vi "1B calc wind acceleration.vi"(8 "Sail Position":dbl, 9 "time elapsed since last iteration":dbl, 10 "Apparent Wind Speed in":T2, 11 "Absolute Wind\nDirection":T1) -> (3 "Wind dV":T2)   [LabVIEW 2011]
doc: "Calculates velocity from the wind. Uses the apparent wind direction and sail angle to determine the fraction of the wind speed we can go at, using several equations that roughly model boat speed, and then multiplies the wind speed by that fraction.\nTODO: currently only does acceleration in the forward direction. should be upgraded to have a side force as well, which can be balanced by a hydrodynamic side force."
uses:
  2-Think/2 Typedefs/apparent wind speed.ctl
  2-Think/2 Typedefs/apparent wind direction.ctl
  2-Think/2 Typedefs/heading.ctl
  2-Think/2 Globals/2 TuningConstants.vi
  2-Think/2 Globals/2 Global.vi
panel:
  out "In Irons?":bool
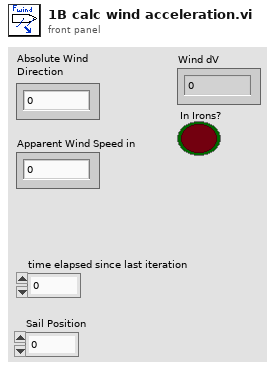
[diagram p1: front panel]
types:
  T1 = typedef "apparent wind direction.ctl" = dbl
  T2 = typedef "apparent wind speed.ctl" = dbl
  T3 = typedef "heading.ctl" = dbl
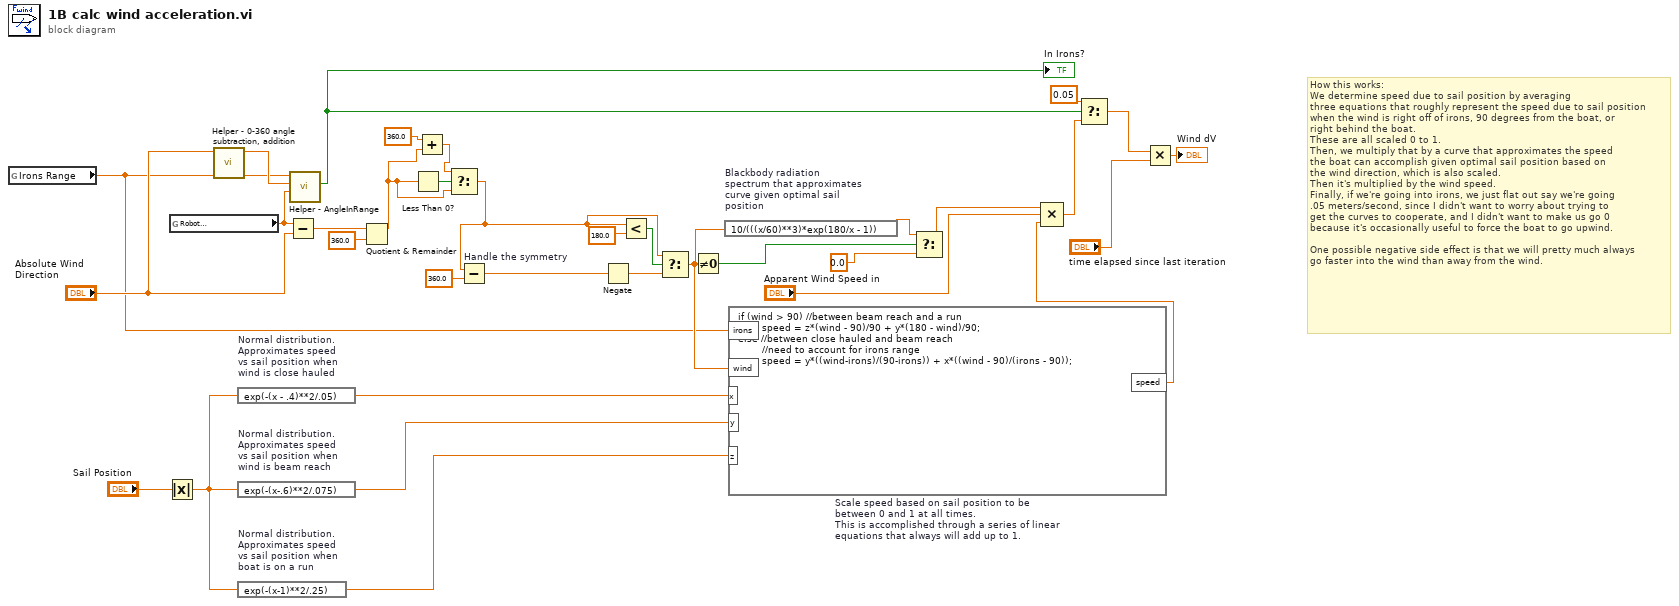
[diagram p0: block diagram]
diagram:
  # "How this works:\nWe determine speed due to sail position by averaging\nthree equations that roughly represent the speed due to sail position\nwhen the wind is right off of irons, 90 degrees from the boat, or\nright behind the boat.\nThese are all scaled 0 to 1.\nThen, we multiply that by a curve that approximates the speed\nthe boat can accomplish given optimal sail position based on\nthe wind direction, which is also scaled.\nThen it's multiplied by the wind speed.\nFinally, if we're going into irons, we just flat out say we're going\n.05 meters/second, since I didn't want to worry about trying to\nget the curves to cooperate, and I didn't want to make us go 0\nbecause it's occasionally useful to force the boat to go upwind.\n\nOne possible negative side effect is that we will pretty much always\ngo faster into the wind than away from the wind."
  n1 = global read "2 TuningConstants.vi" "Irons Range"() -> (w5:dbl)
  n2 = Absolute Value(x="Sail Position") -> (abs(x)=w1:dbl)
  n3 = global read "2 Global.vi" "Robot\nHeading"() -> (w15:T3)
  n4 = call "Helper - 0-360 angle subtraction, addition.vi"("y"=w5, "x"="Absolute Wind\nDirection") -> ("x + y"=w3:dbl, "x - y"=w4:T1)  [unwired: 8 in]
  n5 = expression code="exp(-(x - .4)**2/.05)" "Normal distribution.\nApproximates speed \nvs sail position when\nwind is close hauled"(w1) -> (w24:dbl)
  n6 = expression code="exp(-(x-.6)**2/.075)" "Normal distribution.\nApproximates speed\nvs sail position when\nwind is beam reach"(w1) -> (w23:dbl)
  n7 = expression code="exp(-(x-1)**2/.25)" "Normal distribution.\nApproximates speed\nvs sail position when\nboat is on a run"(w1) -> (w22:dbl)
  n8 = Subtract(x=w15, y="Absolute Wind\nDirection") -> (x-y=w12:T3)
  n9 = call "Helper - AngleInRange.vi"("Angle to check"=w15, "Angle 2"=w4, "Angle 1"=w3) -> ("In range?"=w14:bool)  [unwired: 8 in]
  "In Irons?" <- w14
  n10 = Quotient & Remainder(x=w12, y=T3 360.0) -> (x-y*floor(x/y)=w7:T3)  [unwired: 1 out]
  n11 = Less Than 0?(x=w7) -> (x < 0?=w10:bool)
  n12 = Add(x=T3 360.0, y=w7) -> (x+y=w8:T3)
  n13 = Select(t=w8, s=w10, f=w7) -> (s? t:f=w9:T3)
  n14 = Subtract "Handle the symmetry"(x=w9, y=T1 360.0) -> (x-y=w25:T3)
  n15 = Negate(x=w25) -> (-x=w26:T3)
  n16 = Less?(x=w9, y=T1 180.0) -> (x < y?=w28:bool)
  n17 = Select(t=w9, s=w28, f=w26) -> (s? t:f=w17:T3)
  n18 = Not Equal To 0?(x=w17) -> (x != 0?=w16:bool)
  n19 = expression code="10/(((x/60)**3)*exp(180/x - 1))" "Blackbody radiation\nspectrum that approximates\ncurve given optimal sail\nposition"(w17) -> (w20:T3)
  n20 = formula code="if (wind > 90) //between beam reach and a run\n        speed = z*(wind - 90)/90 + y*(180 - wind)/90;\nelse //between close hauled and beam reach\n        //need to account for irons range\n        speed = y*((wind-irons)/(90-irons)) + x*((wind - 90)/(irons - 90));" "Scale speed based on sail position to be between 0 and 1 at all times.\nThis is accomplished through a series of linear equations that always will add up to 1."("x"=w24, "y"=w23, "z"=w22, "wind"=w17, "irons"=w5) -> ("speed"=w21:dbl)
  n21 = Select(t=w20, s=w16, f=T1 0.0) -> (s? t:f=w18:T1)
  n22 = Compound Arithmetic op=MULTIPLY(w18, "Apparent Wind Speed in", w21) -> (w31:T1)
  n23 = Select(t=T2 0.05 ("Apparent Wind Speed"), s=w14, f=w31) -> (s? t:f=w35:T1)
  n24 = Multiply(x=w35, y="time elapsed since last iteration") -> (x*y=→"Wind dV":T1)
